vi "Auto Trader.vi"(9 "Pages to Pull":i32, 10 "Link":string="https://www.autotrader.co.uk/car-search?postcode=MK8%200BS&price-to=3000&include-delivery-option=on&onesearchad=Used&onesearchad=Nearly%20New&onesearchad=New&advertising-location=at_cars&page=") -> (2 "Pulled Cars":string[][](array[string]), 3 "Car Information":string[][](array[string]))   [LabVIEW 2018]
uses:
  e746313a-f7cd-4b2e-8300-9873ca4d51e3.vi
  <vilib>/Array/Sort 2D Array - Pop Stack.vi
  <vilib>/Array/Sort 2D Array - Push Stack.vi
  <vilib>/httpClient/LabVIEWHTTPClient.lvlib
  <vilib>/gmath/NI_Gmath.lvlib
panel:
  out "Page No.":i32
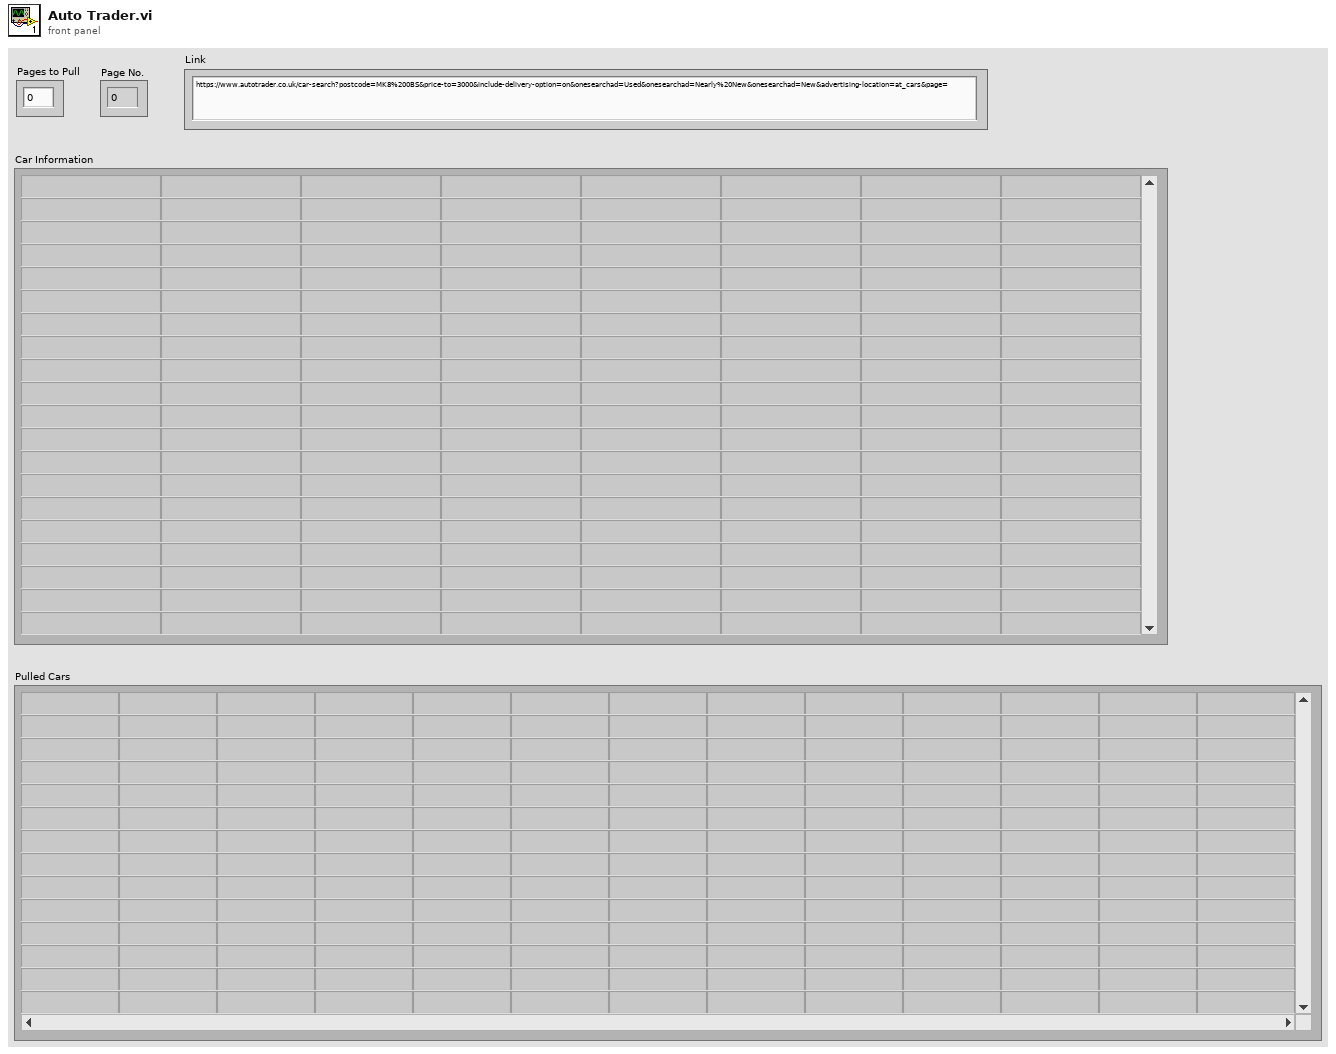
[diagram p1: front panel]
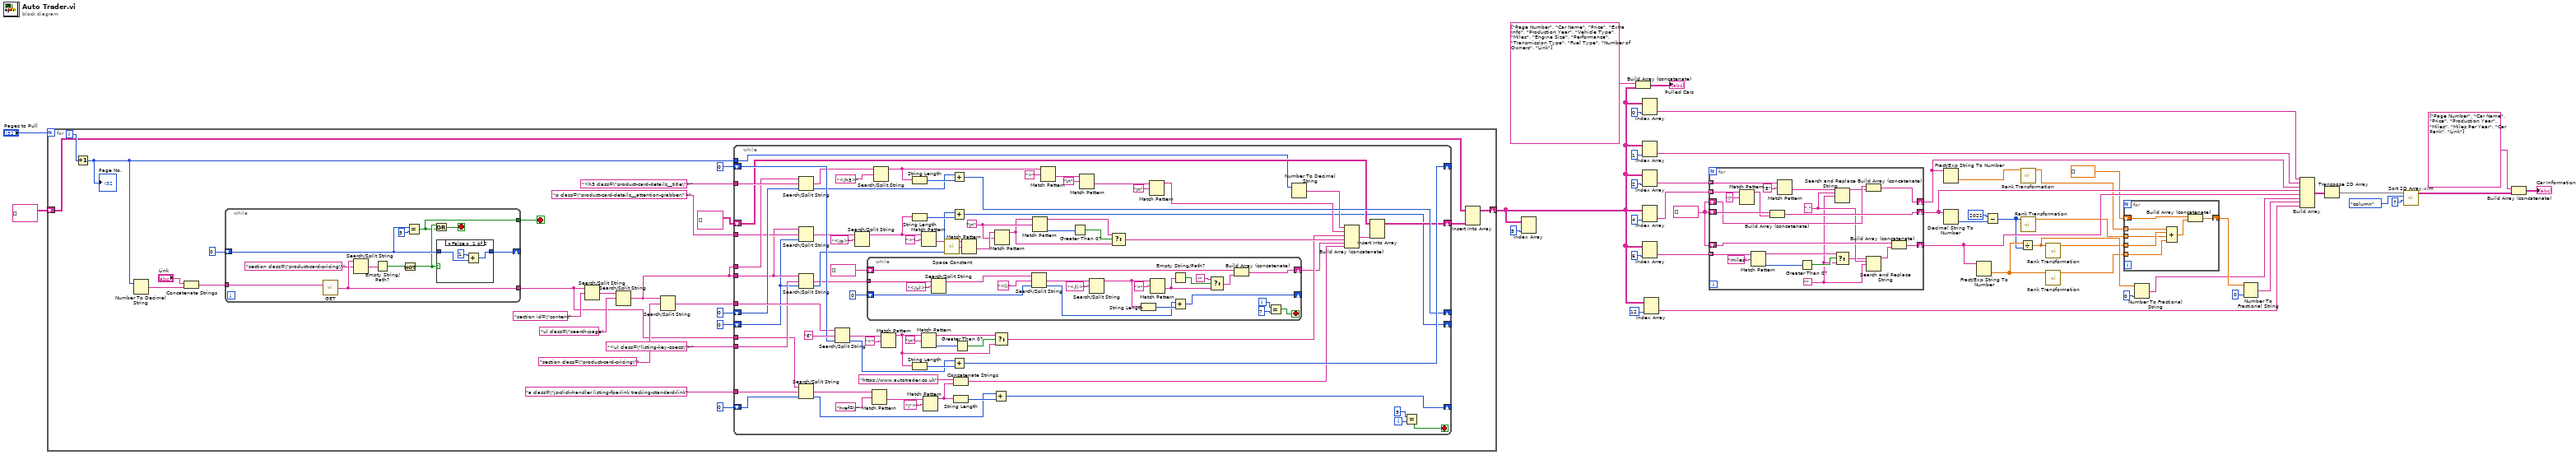
[diagram p0: block diagram]
diagram:
  w26 = string[] []
  n1 = for {
    N: "Pages to Pull" -> [_]
    shift-right: [w57] -> w8
    shift-left: string[][] [] -> [w56]
    i -> [w66]
    stop <- w50 stop-if-true
    n2 = Increment(x=w66) -> (x+1=w48:i32)
    "Page No." <- w48
    n3 = Number To Decimal String(number=w48) -> (decimal integer string=w65:string)  [unwired: 1 in]
    n4 = Concatenate Strings("Link", w65) -> (w64:string)
    n5 = while {
      tunnel: w64 -> [w82]
      tunnel: [w81] -> w52
      shift-right: [w77] -> _
      shift-left: 0 -> [w76]
      tunnel: [w72] -> w50
      stop <- w73 stop-if-true
      n6 = call <vilib>:"GET.vi"("url"=w82) -> ("body"=w81:string)  [unwired: 11 in, 3 out]
      n7 = Search/Split String(string=w81, search string/char (-)="section class=\"product-card-pricing\"") -> (match + rest of string=w79:string)  [unwired: 1 in, 2 out]
      n8 = Empty String/Path?(string/path=w79) -> (empty?=w78:bool)
      n9 = Not(x=w78) -> (.not. x?=w74:bool)
      n10 = Equal?(x=w76, y=5) -> (x = y?=w72:bool)
      n11 = Or(x=w74, y=w72) -> (x .or. y?=w73:bool)
      n12 = case shown="False" w74 {
        tunnel: [w83 w86] -> w77
        tunnel: w76 -> [w84 w86]
        frame False {
          n13 = Add(x=1, y=w84) -> (x+y=w83:i32)
        }
        frame True {
        }
      }
    }
    n14 = Search/Split String(string=w52, search string/char (-)="section id=\"content") -> (match + rest of string=w53:string)  [unwired: 1 in, 2 out]
    n15 = Search/Split String(string=w53, search string/char (-)="ul class=\"search-page") -> (match + rest of string=w47:string)  [unwired: 1 in, 2 out]
    n16 = Search/Split String(string=w47, search string/char (-)="section class=\"product-card-pricing\"") -> (match + rest of string=w68:string)  [unwired: 1 in, 2 out]
    n17 = while {
      shift-right: [w158] -> _
      shift-left: 0 -> [w156]
      tunnel: w68 -> [w154]
      shift-right: [w134] -> w58
      shift-left: string[][] [] -> [w135]
      shift-right: [w146] -> _
      shift-left: 0 -> [w138]
      shift-right: [w92] -> _
      shift-left: 0 -> [w87]
      tunnel: "<h3 class=\"product-card-details__title\">" ("search string/char (-)") -> [w143]
      tunnel: w47 -> [w142]
      tunnel: "<ul class=\"listing-key-specs\">" -> [w140]
      tunnel: w47 -> [w90]
      tunnel: "a class=\"js-click-handler listing-fpa-link tracking-standard-link" ("search string/char (-)") -> [w130]
      tunnel: w52 -> [w129]
      shift-right: [w122] -> _
      shift-left: 0 -> [w126]
      tunnel: w48 -> [w116]
      tunnel: "p class=\"product-card-details__attention-grabber\">" ("search string/char (-)") -> [w91]
      i -> [w96]
      stop <- w95 stop-if-true
      w107 = "\n"
      n18 = Search/Split String(string=w142, search string/char (-)=w143, offset (0)=w138) -> (match + rest of string=w141:string, offset of match=w137:i32)  [unwired: 1 out]
      n19 = Search/Split String(string=w90, search string/char (-)=w91, offset (0)=w87) -> (match + rest of string=w89:string)  [unwired: 2 out]
      n20 = Search/Split String(string=w90, search string/char (-)=w140, offset (0)=w87) -> (match + rest of string=w88:string, offset of match=w139:i32)  [unwired: 1 out]
      n21 = Search/Split String(string=w129, search string/char (-)=w130, offset (0)=w126) -> (match + rest of string=w121:string, offset of match=w123:i32)  [unwired: 1 out]
      n22 = Search/Split String(string=w154, search string/char (-)="£", offset (0)=w156) -> (match + rest of string=w131:string, offset of match=w157:i32)  [unwired: 1 out]
      n23 = Search/Split String(string=w89, search string/char (-)="</p>") -> (substring before match=w144:string)  [unwired: 1 in, 2 out]
      n24 = while {
        tunnel: w88 -> [w171]
        shift-right: [w175] -> _
        shift-left: 0 -> [w178]
        shift-right: [w174] -> w93
        shift-left: string[] [] -> [w173]
        i -> [w163]
        stop <- w161 stop-if-true
        n25 = Search/Split String(string=w171, search string/char (-)="</ul>") -> (substring before match=w164:string)  [unwired: 1 in, 2 out]
        n26 = Search/Split String(string=w164, search string/char (-)="<li", offset (0)=w178) -> (match + rest of string=w169:string, offset of match=w176:i32)  [unwired: 1 out]
        n27 = Search/Split String(string=w169, search string/char (-)="</li>" ("regular expression")) -> (substring before match=w172:string)  [unwired: 1 in, 2 out]
        n28 = String Length(string=w172) -> (length=w177:i32)
        n29 = Match Pattern(string=w172, regular expression=">") -> (after substring=w166:string)  [unwired: 1 in, 3 out]
        n30 = Empty String/Path?(string/path=w166) -> (empty?=w168:bool)
        n31 = Add(x=w176, y=w177) -> (x+y=w175:i32)
        n32 = Select(t="", s=w168, f=w166) -> (s? t:f=w165:string)
        n33 = Build Array (concatenate)(w173, w165) -> (w174:string[])
        n34 = Equal?(x=w163, y=7) -> (x = y?=w161:bool)
      }
      n35 = Match Pattern(string=w121, regular expression="href=\"" ("search string/char (-)")) -> (after substring=w124:string)  [unwired: 1 in, 3 out]
      n36 = Search/Split String(string=w141, search string/char (-)="</h3>") -> (substring before match=w147:string)  [unwired: 1 in, 2 out]
      n37 = Match Pattern(string=w131, regular expression="<" ("search string/char (-)")) -> (before substring=w100:string)  [unwired: 1 in, 3 out]
      n38 = String Length(string=w147) -> (length=w148:i32)
      n39 = String Length(string=w144) -> (length=w145:i32)
      n40 = String Length(string=w100) -> (length=w159:i32)
      n41 = Match Pattern(string=w144, regular expression=">") -> (after substring=w133:string)  [unwired: 1 in, 3 out]
      n42 = Match Pattern(string=w100, regular expression="\n") -> (before substring=w98:string, offset past match=w102:i32)  [unwired: 1 in, 2 out]
      n43 = Match Pattern(string=w124, regular expression="\">") -> (before substring=w118:string)  [unwired: 1 in, 3 out]
      n44 = call <vilib>:"Space Constant.vi"() -> ("String"=w115:string)
      n45 = Add(x=w137, y=w148) -> (x+y=w146:i32)
      n46 = Add(x=w139, y=w145) -> (x+y=w92:i32)
      n47 = Add(x=w157, y=w159) -> (x+y=w158:i32)
      n48 = Concatenate Strings("https://www.autotrader.co.uk" ("string"), w118) -> (w119:string)
      n49 = String Length(string=w118) -> (length=w125:i32)
      n50 = Greater Than 0?(x=w102) -> (x > 0?=w101:bool)
      n51 = Match Pattern(string=w133, regular expression=w115) -> (after substring=w109:string)  [unwired: 1 in, 3 out]
      n52 = Add(x=w123, y=w125) -> (x+y=w122:i32)
      n53 = Match Pattern(string=w109, regular expression=w107) -> (before substring=w105:string)  [unwired: 1 in, 3 out]
      n54 = Select(t=w98, s=w101, f=w100) -> (s? t:f=w99:string)
      n55 = Match Pattern(string=w105, regular expression=w107) -> (before substring=w97:string, offset past match=w106:i32)  [unwired: 1 in, 2 out]
      n56 = Match Pattern(string=w147, regular expression=">" ("search string/char (-)")) -> (after substring=w113:string)  [unwired: 1 in, 3 out]
      n57 = Greater Than 0?(x=w106) -> (x > 0?=w108:bool)
      n58 = Match Pattern(string=w113, regular expression="\n") -> (after substring=w111:string)  [unwired: 1 in, 3 out]
      n59 = Select(t=w97, s=w108, f=w105) -> (s? t:f=w104:string)
      n60 = Match Pattern(string=w111, regular expression="\n") -> (before substring=w110:string)  [unwired: 1 in, 3 out]
      n61 = Number To Decimal String(number=w116) -> (decimal integer string=w117:string)  [unwired: 1 in]
      n62 = Build Array (concatenate)(w117, w110, w99, w104, w93, w119) -> (w136:string[])
      n63 = Insert Into Array(array=w135, new element=w136) -> (w134:string[][])  [unwired: 2 in]
      n64 = Equal?(x=9, y=w96) -> (x = y?=w95:bool)
    }
    n65 = Insert Into Array(array=w56, new element=w58) -> (w57:string[][])  [unwired: 2 in]
  }
  n66 = Index Array(array=w8, index (col)=5) -> ()  [unwired: 1 in, 1 out]
  n67 = Build Array (concatenate)(string[] ["Page Number", "Car Name", "Price", "Extra Info", "Production Year", "Vehicle Type", "Miles", "Engine Size", "Performance", "Transmission Type", "Fuel Type", "Number of Owners", "Link"], w8) -> (→"Pulled Cars":string[][])
  n68 = Index Array(array=w8, index (col)=0 ("disabled index (col)")) -> (element=w25:string[])  [unwired: 1 in]
  n69 = Index Array(array=w8, index (col)=1 ("disabled index (col)")) -> (element=w6:string[])  [unwired: 1 in]
  n70 = Index Array(array=w8, index (col)=2) -> (element=w27:string[])  [unwired: 1 in]
  n71 = Index Array(array=w8, index (col)=4 ("disabled index (col)")) -> (element=w40:string[])  [unwired: 1 in]
  n72 = Index Array(array=w8, index (col)=6 ("disabled index (col)")) -> (element=w38:string[])  [unwired: 1 in]
  n73 = Index Array(array=w8, index (col)=12) -> (element=w7:string[])  [unwired: 1 in]
  n74 = for {
    tunnel: w40 -> [w203] mode=indexing
    shift-right: [w201] -> w32
    shift-left: w26 -> [w200]
    tunnel: w38 -> [w198] mode=indexing
    shift-right: [w196] -> w33
    shift-left: w26 -> [w195]
    tunnel: w27 -> [w193] mode=indexing
    shift-right: [w192] -> w24
    shift-left: w26 -> [w191]
    w188 = "," ("search string")
    w183 = ""
    n75 = Match Pattern(string=w203, regular expression="(") -> (before substring=w199:string)  [unwired: 1 in, 3 out]
    n76 = Match Pattern(string=w198, regular expression="miles") -> (before substring=w184:string, offset past match=w185:i32)  [unwired: 1 in, 2 out]
    n77 = Build Array (concatenate)(w200, w199) -> (w201:string[])
    n78 = Match Pattern(string=w193, regular expression="£") -> (after substring=w190:string)  [unwired: 1 in, 3 out]
    n79 = Greater Than 0?(x=w185) -> (x > 0?=w186:bool)
    n80 = Search and Replace String(input string=w190, search string=w188, replace string=w183) -> (result string=w189:string)  [unwired: 5 in, 3 out]
    n81 = Select(t=w184, s=w186, f=w183) -> (s? t:f=w182:string)
    n82 = Build Array (concatenate)(w191, w189) -> (w192:string[])
    n83 = Search and Replace String(input string=w182, search string=w188, replace string=w183) -> (result string=w187:string)  [unwired: 5 in, 3 out]
    n84 = Build Array (concatenate)(w195, w187) -> (w196:string[])
  }
  n85 = Fract/Exp String To Number(string=w24) -> (number=w23:dbl[])  [unwired: 3 in, 1 out]
  n86 = Decimal String To Number(string=w32) -> (number=w30:i32[])  [unwired: 2 in, 1 out]
  n87 = Fract/Exp String To Number(string=w33) -> (number=w22:dbl[])  [unwired: 3 in, 1 out]
  n88 = Subtract(x=2021, y=w30) -> (x-y=w2:i32[])
  n89 = Divide(x=w22, y=w2) -> (x/y=w21:dbl[])
  n90 = call <vilib>:"Rank Transformation.vi"("x"=w23) -> ("rank order x"=w1:dbl[])  [unwired: 9 in, 1 out]
  n91 = call <vilib>:"Rank Transformation.vi"("x"=w2) -> ("rank order x"=w3:dbl[])  [unwired: 9 in, 1 out]
  n92 = call <vilib>:"Rank Transformation.vi"("x"=w21) -> ("rank order x"=w4:dbl[])  [unwired: 9 in, 1 out]
  n93 = call <vilib>:"Rank Transformation.vi"("x"=w22) -> ("rank order x"=w5:dbl[])  [unwired: 9 in, 1 out]
  n94 = for {
    tunnel: w1 -> [w204] mode=indexing
    tunnel: w4 -> [w210] mode=indexing
    tunnel: w3 -> [w209] mode=indexing
    tunnel: w5 -> [w208] mode=indexing
    shift-right: [w207] -> w13
    shift-left: dbl[] [] -> [w206]
    n95 = Compound Arithmetic op=ADD(w204, w210, w209, w208) -> (w205:dbl)
    n96 = Build Array (concatenate)(w206, w205) -> (w207:dbl[])
  }
  n97 = Number To Fractional String(number=w21, precision (6)=i16 0) -> (F-format string=w11:string[])  [unwired: 2 in]
  n98 = Number To Fractional String(number=w13, precision (6)=i16 0) -> (F-format string=w10:string[])  [unwired: 2 in]
  n99 = Build Array(w25, w6, w24, w32, w33, w11, w10, w7) -> (w36:string[][])
  n100 = Transpose 2D Array(2D array=w36) -> (transposed array=w18:string[][])
  n101 = call "Sort 2D Array.vim"("index"=7, "dimension to index (column)"=enum16{"column", "row"}."column", "2D array"=w18) -> ("sorted 2D array"=w17:string[][])  [unwired: 7 in, 1 out]
  n102 = Build Array (concatenate)(string[] ["Page Number", "Car Name", "Price", "Production Year", "Miles", "Miles Per Year", "Car Rank", "Link"], w17) -> (→"Car Information":string[][])
